vi "Circle_Wizard.vi"(9 "Piezo in":refnum<visa-resource-name>, 10 "XY in":refnum<visa-resource-name>, 11 "Coordinates in":dbl[][](array[numeric])) -> (3 "Coordinates out":dbl[][](array[numeric]))   [LabVIEW 2015]
panel:
  in  "9":bool
  in  "8":bool
  in  "7":bool
  in  "6":bool
  in  "5":bool
  in  "4":bool
  in  "3":bool
  in  "2":bool
  in  "1":bool
  in  "Load parameter":bool
  in  "Cancel Button":bool
  in  "OK Button":bool
  in  "Parameter values":dbl[](array[numeric])=[0.0, 0.0, 0.0, 0.0, 0.0, 0.0, 0.0, 0.0, 0.0]
  out "Parameter names":string[](array[string])
  in  "Scan Pattern":T1(radio)
  # "Parameter names"
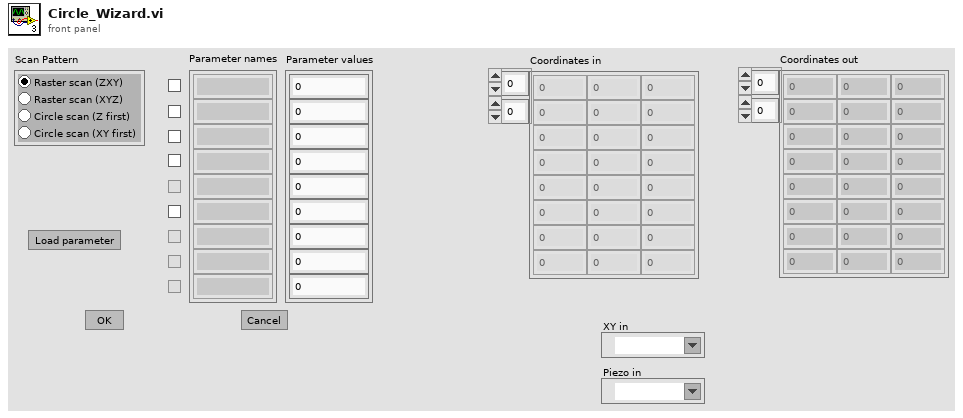
[diagram p1: front panel]
types:
  T1 = enum32{"Raster scan (ZXY)", "Raster scan (XYZ)", "Circle scan (Z first)", "Circle scan (XY first)"}
  T2 = enum8{"Enabled", "Disabled", "Disabled and Grayed Out"}
  T3 = enum16{"Initialize", "Close", "Move Absolute", "Get Position", "Move Relative", "Set Acceleration", "Get Acceleration", "Set Speed", "Get Speed", "Limit Switch Status", "Motor Status", "Stop (controlled)", "Stop (instant)"}
  T4 = enum16{"Initialize", "Close", "Set position", "Get position", "Closed loop on", "Closed loop off", "Remote control on", "Remote control off"}
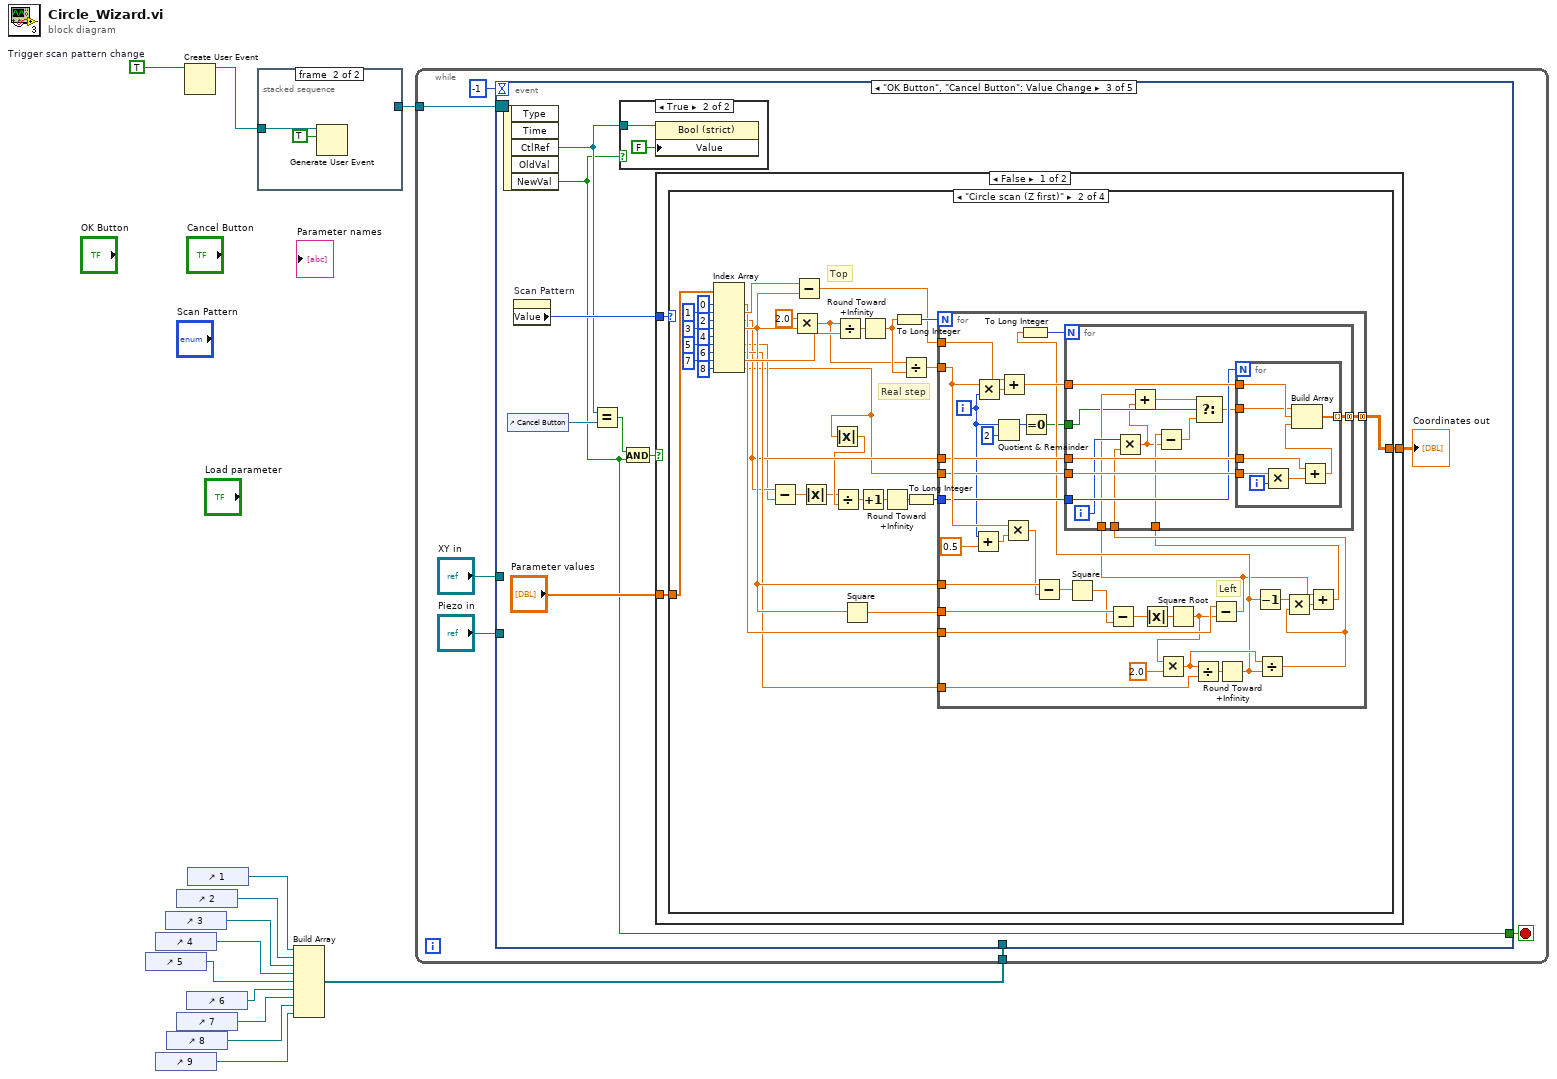
[diagram p0: block diagram]
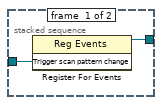
[diagram p2: hidden frame]
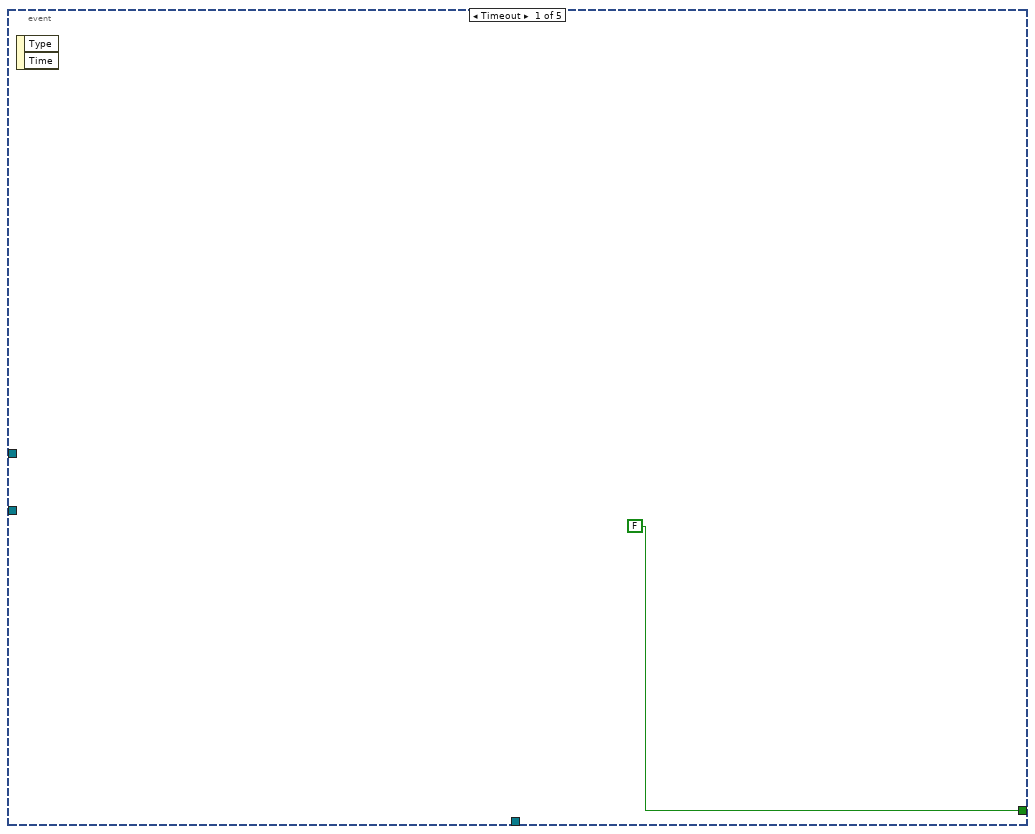
[diagram p3: hidden frame]
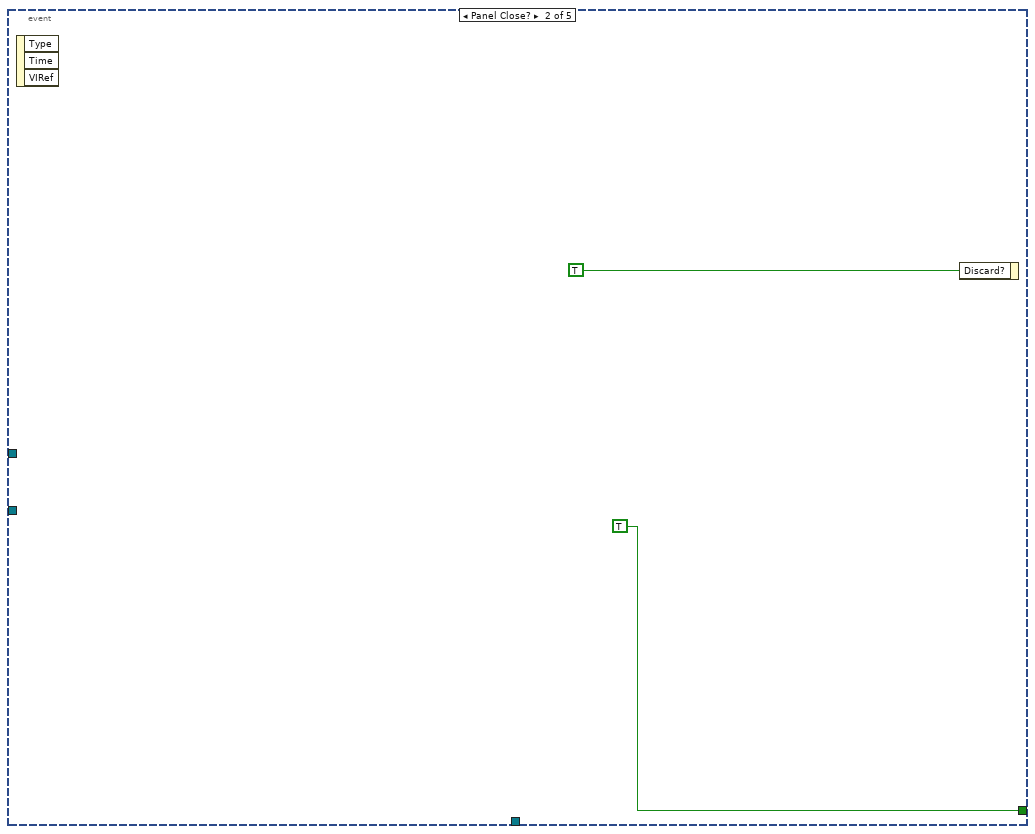
[diagram p4: hidden frame]
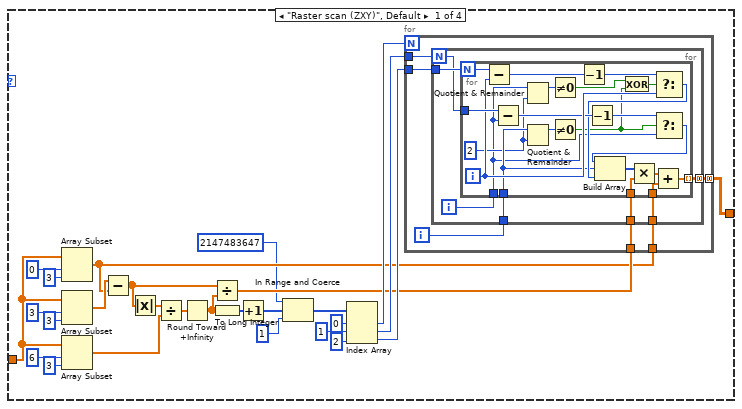
[diagram p6: hidden frame]
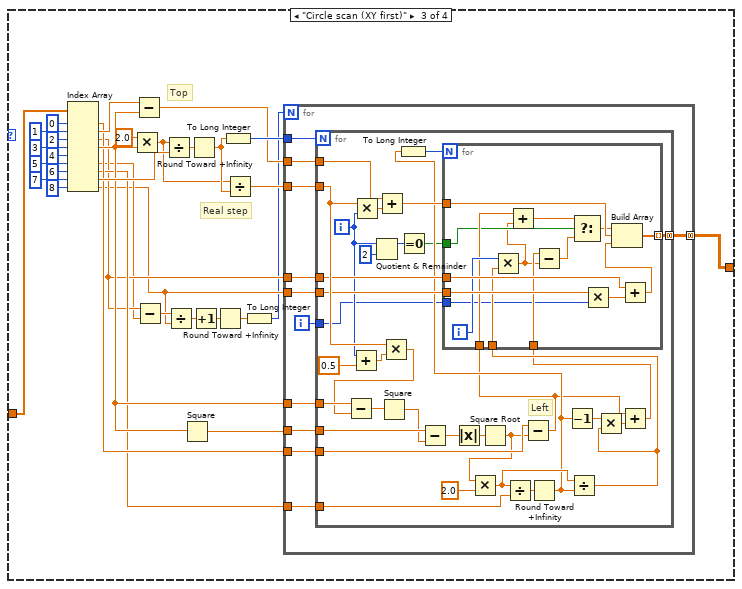
[diagram p7: hidden frame]
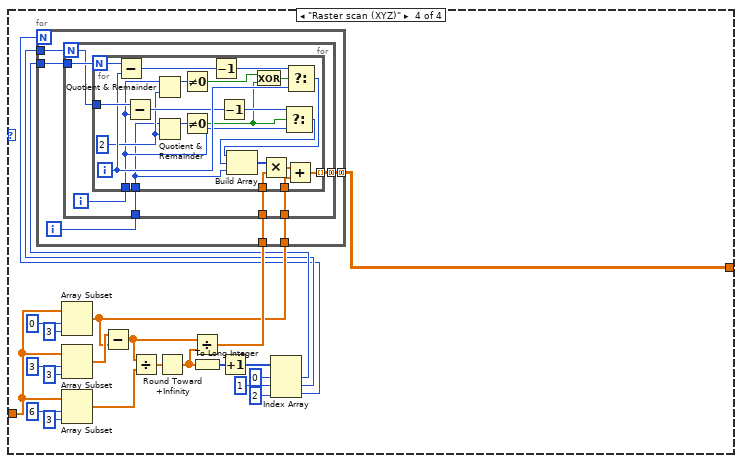
[diagram p8: hidden frame]
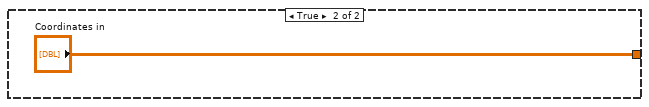
[diagram p9: hidden frame]
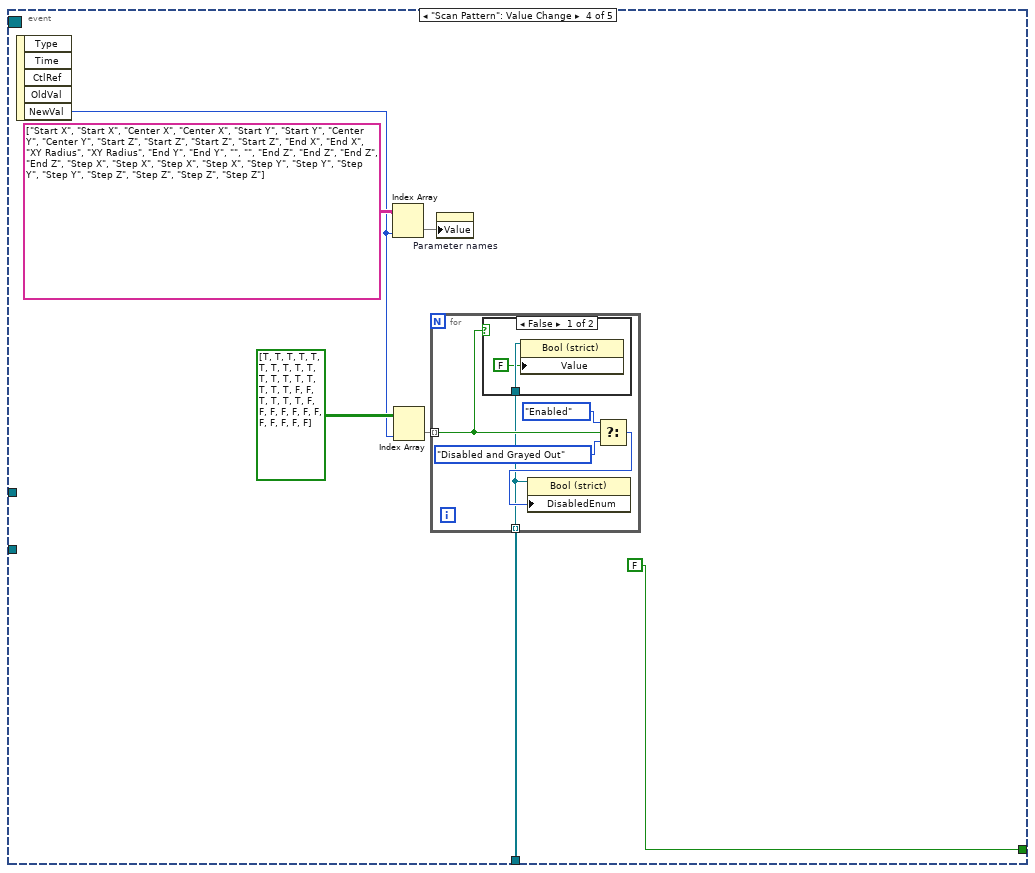
[diagram p10: hidden frame]
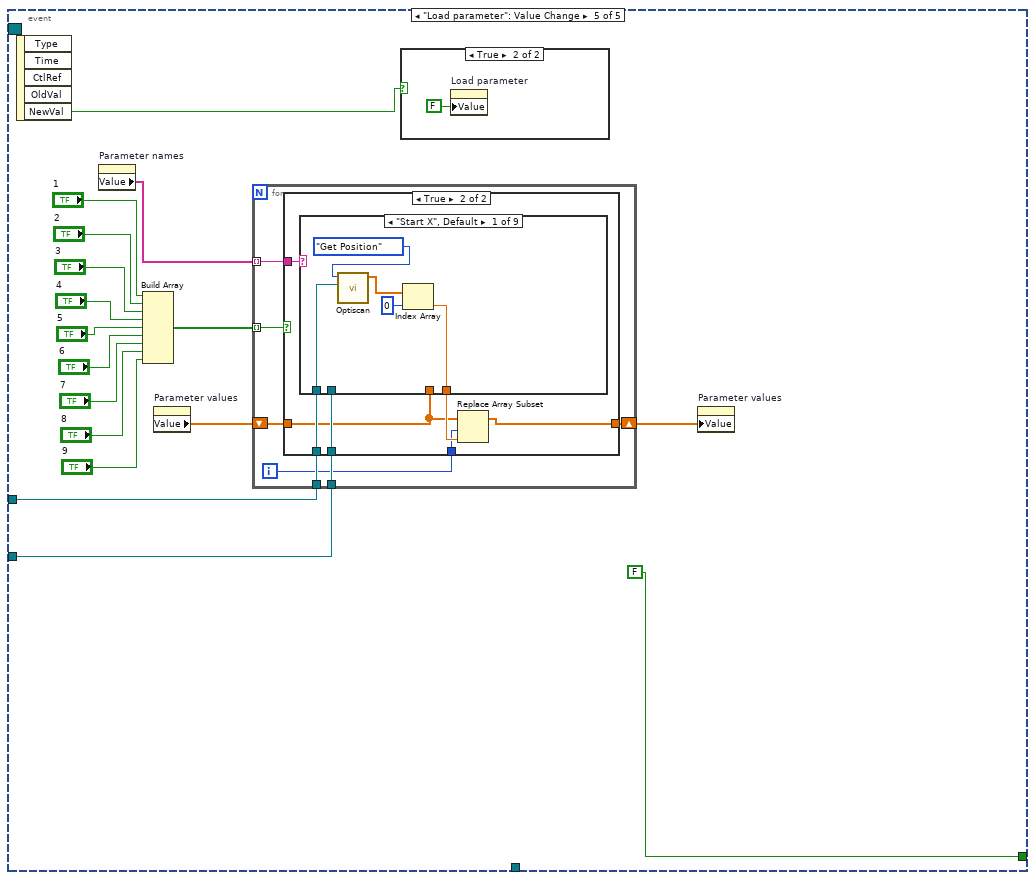
[diagram p12: hidden frame]
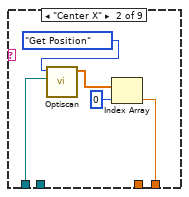
[diagram p15: hidden frame]
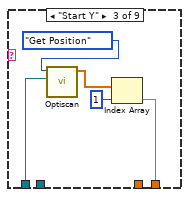
[diagram p16: hidden frame]
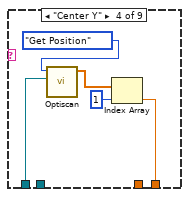
[diagram p17: hidden frame]
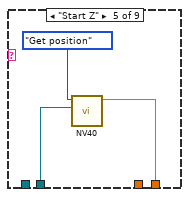
[diagram p18: hidden frame]
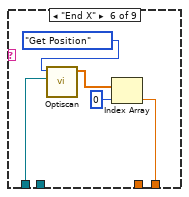
[diagram p19: hidden frame]
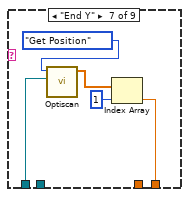
[diagram p20: hidden frame]
diagram:
  w3 = TRUE  # Trigger scan pattern change
  n1 = control-ref of="5"() -> (w9:refnum<vi>)
  n2 = control-ref of="4"() -> (w8:refnum<vi>)
  n3 = control-ref of="9"() -> (w11:refnum<vi>)
  n4 = control-ref of="3"() -> (w7:refnum<vi>)
  n5 = control-ref of="8"() -> (w12:refnum<vi>)
  n6 = control-ref of="2"() -> (w6:refnum<vi>)
  n7 = control-ref of="7"() -> (w13:refnum<vi>)
  n8 = Create User Event(user event datatype=w3) -> (user event=w2:refnum<user-event>)  [unwired: 1 in, 1 out]
  n9 = control-ref of="6"() -> (w10:refnum<vi>)
  n10 = control-ref of="1"() -> (w5:refnum<vi>)
  n11 = stacked-sequence {
    tunnel: w2 -> [w15 w17]
    tunnel: [w14 _] -> w1
    frame #0 {
      n12 = register-events(w15) -> (reference out=w14:refnum<event-registration>)  [unwired: 2 in, 1 out]
    }
    frame #1 {
      n13 = Generate User Event(user event=w17, event data cluster=TRUE ("event data")) -> ()  [unwired: 2 in, 2 out]
    }
  }
  n14 = Build Array(w5, w6, w7, w8, w9, w10, w13, w12, w11) -> (w4:refnum<vi>[])
  n15 = while {
    tunnel: w4 -> [w19]
    tunnel: w1 -> [w18]
    stop <- w23 stop-if-true
    n16 = event shown="[2] \"OK Button\", \"Cancel Button\": Value Change" {
      selector: w18 -> [_ _ _ _ _]
      dyn-events: _ -> [_ _ _ _ _]
      timeout: -1 -> [_ _ _ _ _]
      tunnel: [FALSE TRUE w27 FALSE ("NewVal") FALSE ("NewVal")] -> w23
      tunnel: "XY in" -> [_ _ _ _ w363]
      tunnel: "Piezo in" -> [_ _ _ _ w362]
      tunnel: w19 -> [_ _ _ w344 _]
      event Timeout {
        n17 = event-data() -> ()  [unwired: 1 in, 2 out]
      }
      event Panel Close? {
        n18 = event-data() -> ()  [unwired: 1 in, 3 out]
        n19 = event-data("Discard?"=TRUE) -> ()  [unwired: 1 in, 1 out]
      }
      event "OK Button", "Cancel Button": Value Change {
        n20 = event-data() -> ("CtlRef"=w29:refnum<vi>, "NewVal"=w27:bool)  [unwired: 1 in, 3 out]
        n21 = control-ref of="Cancel Button"() -> (w34:refnum<vi>)
        n22 = property on="Scan Pattern" class="RadioBtnsControl (strict)"() -> ("Value"=w30:T1)  [unwired: 2 in, 2 out]
        n23 = Equal?(x=w29, y=w34) -> (x = y?=w33:bool)
        n24 = case shown="True" w27 {
          tunnel: w29 -> [_ w36]
          frame False {
          }
          frame True {
            n25 = property class="Bool (strict)"(reference=w36, "Value"=FALSE) -> ()  [unwired: 1 in, 2 out]
          }
        }
        n26 = And(x=w33, y=w27) -> (x .and. y?=w32:bool)
        n27 = case shown="False" w32 {
          tunnel: [w37 "Coordinates in"] -> w31
          tunnel: w30 -> [w39 _]
          tunnel: "Parameter values" -> [w38 _]
          frame False {
            n28 = case shown="\"Circle scan (Z first)\"" w39 {
              tunnel: w38 -> [w60 w135 w223 w301]
              tunnel: [w45 w107 w195 w289] -> w37
              frame "Raster scan (ZXY)", Default {
                n29 = Array Subset(array=w60, index=0, length=3) -> (w46:dbl[])
                n30 = Array Subset(array=w60, index=3, length=3) -> (w59:dbl[])
                n31 = Array Subset(array=w60, index=6, length=3) -> (w58:dbl[])
                n32 = Subtract(x=w59, y=w46) -> (x-y=w49:dbl[])
                n33 = Absolute Value(x=w49) -> (abs(x)=w43:dbl[])
                n34 = Divide(x=w43, y=w58) -> (x/y=w57:dbl[])
                n35 = Round Toward +Infinity(x=w57) -> (ceil(x): smallest int >= x=w48:dbl[])
                n36 = Divide(x=w49, y=w48) -> (x/y=w47:dbl[])
                n37 = To Long Integer(number=w48) -> (32bit integer=w56:i32[])
                n38 = Increment(x=w56) -> (x+1=w44:i32[])
                n39 = In Range and Coerce(upper limit=2147483647 ("element"), x=w44, lower limit=1 ("element")) -> (coerced(x)=w42:i32[])  [unwired: 1 out]
                n40 = Index Array(array=w42, index #1=0 ("index"), index #2=1 ("index"), index #3=2 ("index")) -> (element #1=w50:i32, element #2=w51:i32, element #3=w52:i32)
                n41 = for {
                  N: w50 -> [_]
                  tunnel: w52 -> [w72]
                  tunnel: w51 -> [w71]
                  tunnel: w47 -> [w70]
                  tunnel: w46 -> [w69]
                  tunnel: [w68] -> w45 mode=concatenating
                  i -> [w67]
                  n42 = for {
                    N: w71 -> [w73]
                    tunnel: w72 -> [w79]
                    tunnel: w70 -> [w78]
                    tunnel: w69 -> [w77]
                    tunnel: [w76] -> w68 mode=concatenating
                    tunnel: w67 -> [w74]
                    i -> [w75]
                    n43 = for {
                      N: w79 -> [w96]
                      tunnel: w78 -> [w100]
                      tunnel: w77 -> [w98]
                      tunnel: [w97] -> w76 mode=indexing
                      tunnel: w75 -> [w87]
                      tunnel: w74 -> [w89]
                      tunnel: w73 -> [w95]
                      i -> [w94]
                      w88 = 2 ("y")
                      n44 = Subtract(x=w96, y=w94) -> (x-y=w90:i32)
                      n45 = Subtract(x=w95, y=w87) -> (x-y=w93:i32)
                      n46 = Quotient & Remainder(x=w87, y=w88) -> (x-y*floor(x/y)=w85:i32)  [unwired: 1 out]
                      n47 = Quotient & Remainder(x=w89, y=w88) -> (x-y*floor(x/y)=w86:i32)  [unwired: 1 out]
                      n48 = Not Equal To 0?(x=w85) -> (x != 0?=w81:bool)
                      n49 = Not Equal To 0?(x=w86) -> (x != 0?=w80:bool)
                      n50 = Decrement(x=w90) -> (x-1=w84:i32)
                      n51 = Decrement(x=w93) -> (x-1=w83:i32)
                      n52 = Exclusive Or(1:w80, 2:w81) -> (0:w82:bool)
                      n53 = Select(t=w84, s=w82, f=w94) -> (s? t:f=w91:i32)
                      n54 = Select(t=w83, s=w80, f=w87) -> (s? t:f=w92:i32)
                      n55 = Build Array(w92, w89, w91) -> (w101:i32[])
                      n56 = Multiply(x=w101, y=w100) -> (x*y=w99:dbl[])
                      n57 = Add(x=w99, y=w98) -> (x+y=w97:dbl[])
                    }
                  }
                }
              }
              frame "Circle scan (Z first)" {
                # "Real step"
                # "Top"
                n58 = Index Array(array=w135, index #1=0 ("index"), index #2=1 ("index"), index #3=2 ("index"), index #4=3 ("index"), index #5=4 ("index"), index #6=5 ("index"), index #7=6 ("index"), index #8=7 ("index"), index #9=8 ("index")) -> (element #1=w115:dbl, element #2=w120:dbl, element #3=w113:dbl, element #4=w116:dbl, element #6=w112:dbl, element #7=w114:dbl, element #8=w122:dbl, element #9=w104:dbl)  [unwired: 1 out]
                n59 = Subtract(x=w113, y=w112) -> (x-y=w111:dbl)
                n60 = Multiply(x=2.0, y=w116) -> (x*y=w105:dbl)
                n61 = Subtract(x=w120, y=w116) -> (x-y=w119:dbl)
                n62 = Absolute Value(x=w111) -> (abs(x)=w102:dbl)
                n63 = Absolute Value(x=w104) -> (abs(x)=w103:dbl)
                n64 = Divide(x=w102, y=w103) -> (x/y=w110:dbl)
                n65 = Divide(x=w105, y=w122) -> (x/y=w124:dbl)
                n66 = Square(x=w116) -> (x^2=w117:dbl)
                n67 = Increment(x=w110) -> (x+1=w106:dbl)
                n68 = Round Toward +Infinity(x=w124) -> (ceil(x): smallest int >= x=w121:dbl)
                n69 = Round Toward +Infinity(x=w106) -> (ceil(x): smallest int >= x=w109:dbl)
                n70 = To Long Integer(number=w121) -> (32bit integer=w123:i32)
                n71 = Divide(x=w105, y=w121) -> (x/y=w118:dbl)
                n72 = To Long Integer(number=w109) -> (32bit integer=w108:i32)
                n73 = for {
                  N: w123 -> [_]
                  tunnel: w119 -> [w168]
                  tunnel: w118 -> [w163]
                  tunnel: w117 -> [w166]
                  tunnel: w116 -> [w162]
                  tunnel: w115 -> [w149]
                  tunnel: w114 -> [w154]
                  tunnel: w104 -> [w152]
                  tunnel: w113 -> [w151]
                  tunnel: w108 -> [w150]
                  tunnel: [w148] -> w107 mode=concatenating
                  i -> [w144]
                  # "Left"
                  n74 = Add(x=w144, y=0.5) -> (x+y=w164:dbl)
                  n75 = Multiply(x=w163, y=w144) -> (x*y=w169:dbl)
                  n76 = Quotient & Remainder(x=w144, y=2) -> (x-y*floor(x/y)=w142:i32)  [unwired: 1 out]
                  n77 = Add(x=w168, y=w169) -> (x+y=w167:dbl)
                  n78 = Multiply(x=w163, y=w164) -> (x*y=w161:dbl)
                  n79 = Equal To 0?(x=w142) -> (x = 0?=w141:bool)
                  n80 = Subtract(x=w162, y=w161) -> (x-y=w160:dbl)
                  n81 = Square(x=w160) -> (x^2=w159:dbl)
                  n82 = Subtract(x=w166, y=w159) -> (x-y=w158:dbl)
                  n83 = Absolute Value(x=w158) -> (abs(x)=w157:dbl)
                  n84 = Square Root(x=w157) -> (sqrt(x)=w139:dbl)
                  n85 = Multiply(x=w139, y=2.0) -> (x*y=w147:dbl)
                  n86 = Divide(x=w147, y=w154) -> (x/y=w155:dbl)
                  n87 = Subtract(x=w149, y=w139) -> (x-y=w137:dbl)
                  n88 = Round Toward +Infinity(x=w155) -> (ceil(x): smallest int >= x=w145:dbl)
                  n89 = To Long Integer(number=w145) -> (32bit integer=w153:i32)
                  n90 = Decrement(x=w145) -> (x-1=w136:dbl)
                  n91 = Divide(x=w147, y=w145) -> (x/y=w146:dbl)
                  n92 = Multiply(x=w136, y=w146) -> (x*y=w140:dbl)
                  n93 = Add(x=w137, y=w140) -> (x+y=w138:dbl)
                  n94 = for {
                    N: w153 -> [_]
                    tunnel: w167 -> [w183]
                    tunnel: w137 -> [w178]
                    tunnel: w152 -> [w182]
                    tunnel: w151 -> [w181]
                    tunnel: w150 -> [w180]
                    tunnel: [w177] -> w148 mode=concatenating
                    tunnel: w146 -> [w176]
                    tunnel: w141 -> [w173]
                    tunnel: w138 -> [w171]
                    i -> [w179]
                    n95 = Multiply(x=w179, y=w176) -> (x*y=w170:dbl)
                    n96 = Add(x=w178, y=w170) -> (x+y=w175:dbl)
                    n97 = Subtract(x=w171, y=w170) -> (x-y=w172:dbl)
                    n98 = Select(t=w175, s=w173, f=w172) -> (s? t:f=w174:dbl)
                    n99 = for {
                      N: w180 -> [_]
                      tunnel: w183 -> [w191]
                      tunnel: w182 -> [w188]
                      tunnel: w181 -> [w187]
                      tunnel: w174 -> [w185]
                      tunnel: [w184] -> w177 mode=indexing
                      i -> [w190]
                      n100 = Multiply(x=w188, y=w190) -> (x*y=w189:dbl)
                      n101 = Add(x=w187, y=w189) -> (x+y=w186:dbl)
                      n102 = Build Array(w185, w191, w186) -> (w184:dbl[])
                    }
                  }
                }
              }
              frame "Circle scan (XY first)" {
                # "Real step"
                # "Top"
                n103 = Index Array(array=w223, index #1=0 ("index"), index #2=1 ("index"), index #3=2 ("index"), index #4=3 ("index"), index #5=4 ("index"), index #6=5 ("index"), index #7=6 ("index"), index #8=7 ("index"), index #9=8 ("index")) -> (element #1=w203:dbl, element #2=w208:dbl, element #3=w201:dbl, element #4=w204:dbl, element #6=w200:dbl, element #7=w202:dbl, element #8=w210:dbl, element #9=w198:dbl)  [unwired: 1 out]
                n104 = Multiply(x=2.0, y=w204) -> (x*y=w193:dbl)
                n105 = Subtract(x=w208, y=w204) -> (x-y=w207:dbl)
                n106 = Subtract(x=w201, y=w200) -> (x-y=w199:dbl)
                n107 = Divide(x=w193, y=w210) -> (x/y=w212:dbl)
                n108 = Divide(x=w199, y=w198) -> (x/y=w197:dbl)
                n109 = Square(x=w204) -> (x^2=w205:dbl)
                n110 = Round Toward +Infinity(x=w212) -> (ceil(x): smallest int >= x=w209:dbl)
                n111 = Increment(x=w197) -> (x+1=w194:dbl)
                n112 = Round Toward +Infinity(x=w194) -> (ceil(x): smallest int >= x=w196:dbl)
                n113 = To Long Integer(number=w209) -> (32bit integer=w211:i32)
                n114 = Divide(x=w193, y=w209) -> (x/y=w206:dbl)
                n115 = To Long Integer(number=w196) -> (32bit integer=w192:i32)
                n116 = for {
                  N: w192 -> [_]
                  tunnel: w211 -> [w234]
                  tunnel: w207 -> [w233]
                  tunnel: w206 -> [w232]
                  tunnel: w205 -> [w231]
                  tunnel: w204 -> [w230]
                  tunnel: w203 -> [w229]
                  tunnel: w202 -> [w228]
                  tunnel: w201 -> [w227]
                  tunnel: w198 -> [w226]
                  tunnel: [w225] -> w195 mode=concatenating
                  i -> [w224]
                  n117 = for {
                    N: w234 -> [_]
                    tunnel: w233 -> [w267]
                    tunnel: w232 -> [w262]
                    tunnel: w231 -> [w265]
                    tunnel: w230 -> [w261]
                    tunnel: w229 -> [w250]
                    tunnel: w228 -> [w254]
                    tunnel: w226 -> [w252]
                    tunnel: w227 -> [w251]
                    tunnel: [w249] -> w225 mode=concatenating
                    tunnel: w224 -> [w235]
                    i -> [w245]
                    # "Left"
                    n118 = Add(x=w245, y=0.5) -> (x+y=w263:dbl)
                    n119 = Multiply(x=w262, y=w245) -> (x*y=w268:dbl)
                    n120 = Quotient & Remainder(x=w245, y=2) -> (x-y*floor(x/y)=w243:i32)  [unwired: 1 out]
                    n121 = Add(x=w267, y=w268) -> (x+y=w266:dbl)
                    n122 = Multiply(x=w262, y=w263) -> (x*y=w236:dbl)
                    n123 = Subtract(x=w261, y=w236) -> (x-y=w260:dbl)
                    n124 = Square(x=w260) -> (x^2=w259:dbl)
                    n125 = Equal To 0?(x=w243) -> (x = 0?=w242:bool)
                    n126 = Subtract(x=w265, y=w259) -> (x-y=w258:dbl)
                    n127 = Absolute Value(x=w258) -> (abs(x)=w257:dbl)
                    n128 = Square Root(x=w257) -> (sqrt(x)=w240:dbl)
                    n129 = Multiply(x=w240, y=2.0) -> (x*y=w248:dbl)
                    n130 = Divide(x=w248, y=w254) -> (x/y=w255:dbl)
                    n131 = Subtract(x=w250, y=w240) -> (x-y=w238:dbl)
                    n132 = Round Toward +Infinity(x=w255) -> (ceil(x): smallest int >= x=w246:dbl)
                    n133 = To Long Integer(number=w246) -> (32bit integer=w253:i32)
                    n134 = Decrement(x=w246) -> (x-1=w237:dbl)
                    n135 = Divide(x=w248, y=w246) -> (x/y=w247:dbl)
                    n136 = Multiply(x=w237, y=w247) -> (x*y=w241:dbl)
                    n137 = Add(x=w238, y=w241) -> (x+y=w239:dbl)
                    n138 = for {
                      N: w253 -> [_]
                      tunnel: w266 -> [w284]
                      tunnel: w238 -> [w280]
                      tunnel: w252 -> [w283]
                      tunnel: w251 -> [w282]
                      tunnel: [w279] -> w249 mode=indexing
                      tunnel: w247 -> [w278]
                      tunnel: w242 -> [w275]
                      tunnel: w239 -> [w273]
                      tunnel: w235 -> [w269]
                      i -> [w281]
                      n139 = Multiply(x=w281, y=w278) -> (x*y=w272:dbl)
                      n140 = Add(x=w280, y=w272) -> (x+y=w277:dbl)
                      n141 = Subtract(x=w273, y=w272) -> (x-y=w274:dbl)
                      n142 = Select(t=w277, s=w275, f=w274) -> (s? t:f=w276:dbl)
                      n143 = Multiply(x=w283, y=w269) -> (x*y=w271:dbl)
                      n144 = Add(x=w282, y=w271) -> (x+y=w270:dbl)
                      n145 = Build Array(w276, w284, w270) -> (w279:dbl[])
                    }
                  }
                }
              }
              frame "Raster scan (XYZ)" {
                n146 = Array Subset(array=w301, index=0, length=3) -> (w290:dbl[])
                n147 = Array Subset(array=w301, index=3, length=3) -> (w300:dbl[])
                n148 = Array Subset(array=w301, index=6, length=3) -> (w299:dbl[])
                n149 = Subtract(x=w300, y=w290) -> (x-y=w293:dbl[])
                n150 = Divide(x=w293, y=w299) -> (x/y=w298:dbl[])
                n151 = Round Toward +Infinity(x=w298) -> (ceil(x): smallest int >= x=w292:dbl[])
                n152 = Divide(x=w293, y=w292) -> (x/y=w291:dbl[])
                n153 = To Long Integer(number=w292) -> (32bit integer=w297:i32[])
                n154 = Increment(x=w297) -> (x+1=w288:i32[])
                n155 = Index Array(array=w288, index #1=0 ("index"), index #2=1 ("index"), index #3=2 ("index")) -> (element #1=w287:i32, element #2=w286:i32, element #3=w285:i32)
                n156 = for {
                  N: w285 -> [_]
                  tunnel: w287 -> [w313]
                  tunnel: w286 -> [w312]
                  tunnel: w291 -> [w311]
                  tunnel: w290 -> [w310]
                  tunnel: [w309] -> w289 mode=concatenating
                  i -> [w308]
                  n157 = for {
                    N: w312 -> [w314]
                    tunnel: w313 -> [w320]
                    tunnel: w311 -> [w319]
                    tunnel: w310 -> [w318]
                    tunnel: [w317] -> w309 mode=concatenating
                    tunnel: w308 -> [w315]
                    i -> [w316]
                    n158 = for {
                      N: w320 -> [w337]
                      tunnel: w319 -> [w341]
                      tunnel: w318 -> [w339]
                      tunnel: [w338] -> w317 mode=indexing
                      tunnel: w316 -> [w331]
                      tunnel: w315 -> [w321]
                      tunnel: w314 -> [w336]
                      i -> [w335]
                      w332 = 2 ("y")
                      n159 = Subtract(x=w337, y=w335) -> (x-y=w333:i32)
                      n160 = Subtract(x=w336, y=w331) -> (x-y=w334:i32)
                      n161 = Quotient & Remainder(x=w331, y=w332) -> (x-y*floor(x/y)=w329:i32)  [unwired: 1 out]
                      n162 = Quotient & Remainder(x=w321, y=w332) -> (x-y*floor(x/y)=w330:i32)  [unwired: 1 out]
                      n163 = Not Equal To 0?(x=w329) -> (x != 0?=w325:bool)
                      n164 = Not Equal To 0?(x=w330) -> (x != 0?=w324:bool)
                      n165 = Decrement(x=w333) -> (x-1=w328:i32)
                      n166 = Decrement(x=w334) -> (x-1=w327:i32)
                      n167 = Exclusive Or(1:w324, 2:w325) -> (0:w326:bool)
                      n168 = Select(t=w327, s=w324, f=w331) -> (s? t:f=w322:i32)
                      n169 = Select(t=w328, s=w326, f=w335) -> (s? t:f=w323:i32)
                      n170 = Build Array(w323, w322, w321) -> (w342:i32[])
                      n171 = Multiply(x=w342, y=w341) -> (x*y=w340:dbl[])
                      n172 = Add(x=w340, y=w339) -> (x+y=w338:dbl[])
                    }
                  }
                }
              }
            }
          }
          frame True {
          }
        }
        "Coordinates out" <- w31
      }
      event "Scan Pattern": Value Change {
        n173 = event-data() -> ("NewVal"=w346:T1)  [unwired: 1 in, 4 out]
        n174 = Index Array(array=string[][] [["Start X", "Start X", "Center X", "Center X"], ["Start Y", "Start Y", "Center Y", "Center Y"], ["Start Z", "Start Z", "Start Z", "Start Z"], ["End X", "End X", "XY Radius", "XY Radius"], ["End Y", "End Y", "", ""], ["End Z", "End Z", "End Z", "End Z"], ["Step X", "Step X", "Step X", "Step X"], ["Step Y", "Step Y", "Step Y", "Step Y"], ["Step Z", "Step Z", "Step Z", "Step Z"]], index (col)=w346) -> (element=w348:string[])  [unwired: 1 in]
        n175 = Index Array(array=bool[][] [[TRUE, TRUE, TRUE, TRUE], [TRUE, TRUE, TRUE, TRUE], [TRUE, TRUE, TRUE, TRUE], [TRUE, TRUE, TRUE, TRUE], [TRUE, TRUE, FALSE, FALSE], [TRUE, TRUE, TRUE, TRUE], [FALSE, FALSE, FALSE, FALSE], [FALSE, FALSE, FALSE, FALSE], [FALSE, FALSE, FALSE, FALSE]], index (col)=w346) -> (element=w345:bool[])  [unwired: 1 in]
        n176 = for {
          tunnel: w345 -> [w352] mode=indexing
          tunnel: w344 -> [w351] mode=indexing
          n177 = case shown="False" w352 {
            tunnel: w351 -> [w357 _]
            frame False {
              n178 = property class="Bool (strict)"(reference=w357, "Value"=FALSE) -> ()  [unwired: 1 in, 2 out]
            }
            frame True {
            }
          }
          n179 = Select(t=T2."Enabled" ("Disabled"), s=w352, f=T2."Disabled and Grayed Out" ("Disabled")) -> (s? t:f=w353:T2)
          n180 = property class="Bool (strict)"(reference=w351, "DisabledEnum"=w353) -> ()  [unwired: 1 in, 2 out]
        }
        n181 = property on="Parameter names" class="Arr (strict)"("Value"=w348) -> ()  [unwired: 2 in, 2 out]
      }
      event "Load parameter": Value Change {
        n182 = event-data() -> ("NewVal"=w360:bool)  [unwired: 1 in, 4 out]
        n183 = property on="Parameter names" class="Arr (strict)"() -> ("Value"=w364:string[])  [unwired: 2 in, 2 out]
        n184 = Build Array("1", "2", "3", "4", "5", "6", "7", "8", "9") -> (w365:bool[])
        n185 = property on="Parameter values" class="Arr (strict)"() -> ("Value"=w359:dbl[])  [unwired: 2 in, 2 out]
        n186 = for {
          tunnel: w365 -> [w382] mode=indexing
          tunnel: w364 -> [w381] mode=indexing
          tunnel: w363 -> [w380]
          tunnel: w362 -> [w379]
          shift-right: [w376] -> w358
          shift-left: w359 -> [w377]
          i -> [w378]
          n187 = case shown="True" w382 {
            tunnel: w381 -> [_ w390]
            tunnel: w380 -> [_ w389]
            tunnel: w379 -> [_ w388]
            tunnel: w378 -> [_ w386]
            tunnel: w377 -> [w383 w385]
            tunnel: [w383 w384] -> w376
            frame False {
            }
            frame True {
              n188 = case shown="\"Start X\", Default" w390 {
                tunnel: w389 -> [w395 w400 w405 w410 _ w418 w423 _ w437]
                tunnel: w388 -> [_ _ _ _ w412 _ _ w425 _]
                tunnel: [w391 w396 w401 w406 w411 w414 w419 w424 w427] -> w387
                tunnel: w385 -> [_ _ _ _ _ _ _ _ w435]
                frame "Start X", Default {
                  n189 = call "Optiscan.vi"("VISA resource name"=w395, "Command"=T3."Get Position") -> ("Parameter out"=w393:dbl[])  [unwired: 4 in, 2 out]
                  n190 = Index Array(array=w393, index=0) -> (element=w391:dbl)
                }
                frame "Center X" {
                  n191 = call "Optiscan.vi"("VISA resource name"=w400, "Command"=T3."Get Position") -> ("Parameter out"=w398:dbl[])  [unwired: 4 in, 2 out]
                  n192 = Index Array(array=w398, index=0) -> (element=w396:dbl)
                }
                frame "Start Y" {
                  n193 = call "Optiscan.vi"("VISA resource name"=w405, "Command"=T3."Get Position") -> ("Parameter out"=w403:dbl[])  [unwired: 4 in, 2 out]
                  n194 = Index Array(array=w403, index=1) -> (element=w401:dbl)
                }
                frame "Center Y" {
                  n195 = call "Optiscan.vi"("VISA resource name"=w410, "Command"=T3."Get Position") -> ("Parameter out"=w408:dbl[])  [unwired: 4 in, 2 out]
                  n196 = Index Array(array=w408, index=1) -> (element=w406:dbl)
                }
                frame "Start Z" {
                  n197 = call "NV40.vi"("VISA resource name"=w412, "Command"=T4."Get position") -> ("Position out"=w411:dbl)  [unwired: 5 in, 1 out]
                }
                frame "End X" {
                  n198 = call "Optiscan.vi"("VISA resource name"=w418, "Command"=T3."Get Position") -> ("Parameter out"=w416:dbl[])  [unwired: 4 in, 2 out]
                  n199 = Index Array(array=w416, index=0) -> (element=w414:dbl)
                }
                frame "End Y" {
                  n200 = call "Optiscan.vi"("VISA resource name"=w423, "Command"=T3."Get Position") -> ("Parameter out"=w421:dbl[])  [unwired: 4 in, 2 out]
                  n201 = Index Array(array=w421, index=1) -> (element=w419:dbl)
                }
                frame "End Z" {
                  n202 = call "NV40.vi"("VISA resource name"=w425, "Command"=T4."Get position") -> ("Position out"=w424:dbl)  [unwired: 5 in, 1 out]
                }
                frame " XY Radius" {
                  n203 = call "Optiscan.vi"("VISA resource name"=w437, "Command"=T3."Get Position") -> ("Parameter out"=w432:dbl[])  [unwired: 4 in, 2 out]
                  n204 = Array Subset(array=w435, index=0, length=2) -> (w431:dbl[])
                  n205 = Subtract(x=w432, y=w431) -> (x-y=w430:dbl[])
                  n206 = Square(x=w430) -> (x^2=w429:dbl[])
                  n207 = Add Array Elements(numeric array=w429) -> (sum=w428:dbl)
                  n208 = Square Root(x=w428) -> (sqrt(x)=w427:dbl)
                }
              }
              n209 = Replace Array Subset(array=w385, new element=w387, index=w386) -> (w384:dbl[])
            }
          }
        }
        n210 = case shown="True" w360 {
          frame False {
          }
          frame True {
            n211 = property on="Load parameter" class="Bool (strict)"("Value"=FALSE ("Load parameter")) -> ()  [unwired: 2 in, 2 out]
          }
        }
        n212 = property on="Parameter values" class="Arr (strict)"("Value"=w358) -> ()  [unwired: 2 in, 2 out]
      }
    }
  }
